vi "Menu Viewer.vi"() -> ()   [LabVIEW 2019, in "Menu Button.xctl"]
doc: "JSMA Module Template - Top Level UI 0.2.0.4\nRob Humfeld - Jet Engineering\nCopyright (c) 2019, Jet Engineering"
uses:
  Menu Button.xctl
  private/Button Config Cluster STYP.ctl
panel:
  out "Array":string[](array[string])
  out "error out":errorcluster
  in  "Path":path=path "C:/Projects/Emerson-PDLabUpdate/Codeline/Main Codeline/Software/Config Files_Host/MenuConfig.ini"
  in  "Tree":string(tree)
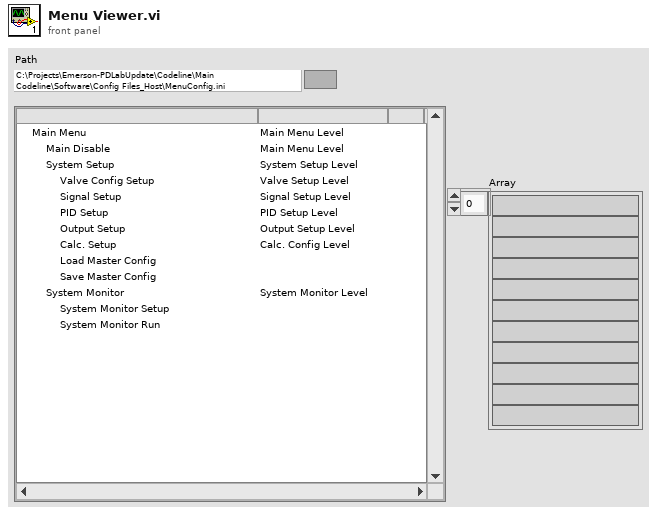
[diagram p1: front panel]
types:
  T1 = typedef "Menu Button.xctl/Button Config Cluster STYP.ctl" = cluster{"ID":string, "Name":string, "Action":string, "Value":string, "Enable?":bool, "Color":string}
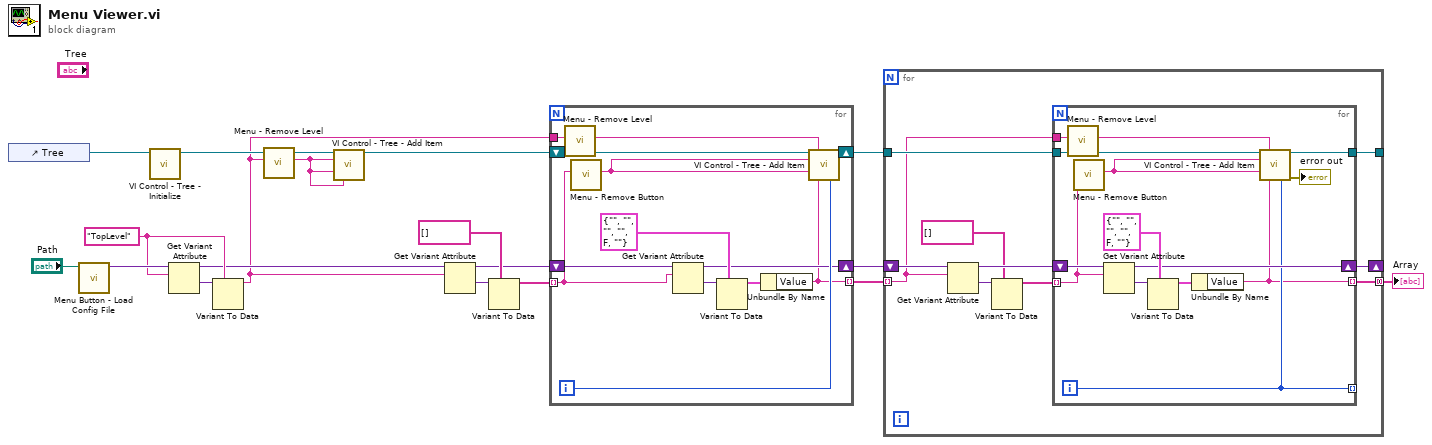
[diagram p0: block diagram]
diagram:
  w14 = "TopLevel" ("name")
  n1 = control-ref of="Tree"() -> (w18:refnum<vi>)
  n2 = call "Menu Button - Load Config File.vi"("Path"="Path") -> ("MenuConfig"=w16:variant)  [unwired: 7 in, 3 out]
  n3 = call <userlib>:"VI Control - Tree - Initialize.vi"("Tree.refnum"=w18) -> ("Tree.refnum"=w13:refnum<vi>)  [unwired: 10 in]
  n4 = Get Variant Attribute(Variant=w16, name=w14) -> (duplicate Variant=w10:variant, value=w15:variant)  [unwired: 2 in, 2 out]
  n5 = Variant To Data(type=w14, Variant=w15) -> (data=w7:string)  [unwired: 1 in, 1 out]
  n6 = call "Menu - Remove Level.vi"("In"=w7) -> ("Out"=w12:string)  [unwired: 10 in]
  n7 = call <userlib>:"VI Control - Tree - Add Item.vi"("Tree.refnum"=w13, "ItemTag"=w12, "ItemLabel"=w12, "ItemText"=w12) -> ("Tree.refnum"=w8:refnum<vi>)  [unwired: 9 in, 2 out]
  n8 = Get Variant Attribute(Variant=w10, name=w7) -> (duplicate Variant=w5:variant, value=w11:variant)  [unwired: 2 in, 2 out]
  n9 = Variant To Data(type=string[] [], Variant=w11) -> (data=w6:string[])  [unwired: 1 in, 1 out]
  n10 = for {
    tunnel: w7 -> [w29]
    tunnel: w6 -> [w20] mode=indexing
    shift-right: [w27] -> w3
    shift-left: w8 -> [w30]
    tunnel: [w19] -> w2 mode=indexing
    shift-right: [w21] -> w4
    shift-left: w5 -> [w24]
    i -> [w26]
    n11 = call "Menu - Remove Level.vi"("In"=w29) -> ("Out"=w28:string)  [unwired: 10 in]
    n12 = call "Menu - Remove Button.vi"("In"=w20) -> ("Out"=w31:string)  [unwired: 10 in]
    n13 = Get Variant Attribute(Variant=w24, name=w20) -> (duplicate Variant=w21:variant, value=w25:variant)  [unwired: 2 in, 2 out]
    n14 = Variant To Data(type=T1 {"ID"="", "Name"="", "Action"="", "Value"="", "Enable?"=FALSE, "Color"=""}, Variant=w25) -> (data=w22:T1)  [unwired: 1 in, 1 out]
    n15 = Unbundle By Name(w22) -> ("Value"=w19:string)
    n16 = call <userlib>:"VI Control - Tree - Add Item.vi"("Tree.refnum"=w30, "Parent Tag"=w28, "Child Position"=w26, "ItemTag"=w31, "ItemLabel"=w31, "ItemText"=w19) -> ("Tree.refnum"=w27:refnum<vi>)  [unwired: 7 in, 2 out]
  }
  n17 = for {
    tunnel: w2 -> [w35] mode=indexing
    tunnel: [w34] -> w1 mode=concatenating
    shift-right: [w32] -> _
    shift-left: w4 -> [w37]
    tunnel: w3 -> [w36]
    tunnel: [w33] -> _
    n18 = Get Variant Attribute(Variant=w37, name=w35) -> (duplicate Variant=w41:variant, value=w38:variant)  [unwired: 2 in, 2 out]
    n19 = Variant To Data(type=string[] [], Variant=w38) -> (data=w40:string[])  [unwired: 1 in, 1 out]
    n20 = for {
      tunnel: w35 -> [w53]
      tunnel: w40 -> [w44] mode=indexing
      tunnel: [w43] -> w34 mode=indexing
      shift-right: [w46] -> w32
      shift-left: w41 -> [w49]
      tunnel: [w45] -> _ mode=indexing
      tunnel: w36 -> [w54]
      tunnel: [w51] -> w33
      i -> [w45]
      n21 = call "Menu - Remove Level.vi"("In"=w53) -> ("Out"=w52:string)  [unwired: 10 in]
      n22 = call "Menu - Remove Button.vi"("In"=w44) -> ("Out"=w55:string)  [unwired: 10 in]
      n23 = Get Variant Attribute(Variant=w49, name=w44) -> (duplicate Variant=w46:variant, value=w50:variant)  [unwired: 2 in, 2 out]
      n24 = Variant To Data(type=T1 {"ID"="", "Name"="", "Action"="", "Value"="", "Enable?"=FALSE, "Color"=""}, Variant=w50) -> (data=w47:T1)  [unwired: 1 in, 1 out]
      n25 = Unbundle By Name(w47) -> ("Value"=w43:string)
      n26 = call <userlib>:"VI Control - Tree - Add Item.vi"("Tree.refnum"=w54, "Parent Tag"=w52, "Child Position"=w45, "ItemTag"=w55, "ItemLabel"=w55, "ItemText"=w43) -> ("Tree.refnum"=w51:refnum<vi>, "error out"=→"error out":errorcluster)  [unwired: 7 in, 1 out]
    }
  }
  "Array" <- w1
